vi "Read configuration.vi"(8 "error in":errorcluster, 11 "cfg group in":refnum<class "group node.lvclass">) -> (0 "error out":errorcluster, 2 "configuration":refnum<class "NISE_CEF_serializable configuration.lvclass">, 3 "cfg group out":refnum<class "group node.lvclass">)   [LabVIEW 2014, in "group node.lvclass"]
uses:
  group node.lvclass
  <vilib>/NI/Configuration Framework/serializable configuration/NISE_CEF_serializable configuration.lvclass
  group node.lvclass/group node.ctl
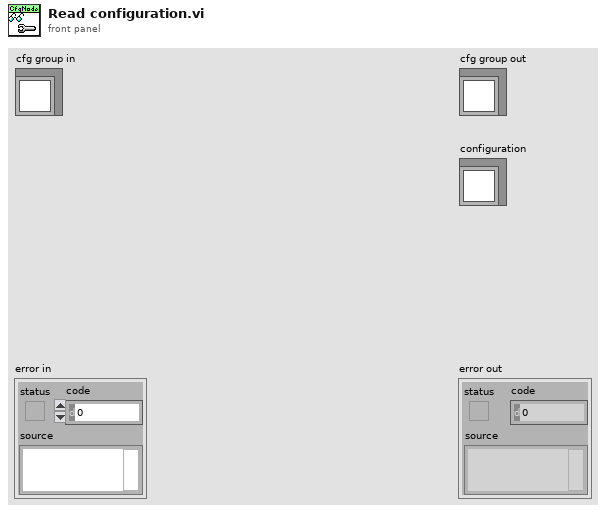
[diagram p1: front panel]
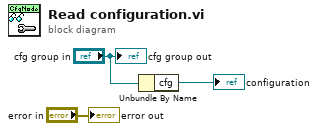
[diagram p0: block diagram]
diagram:
  n1 = Unbundle By Name("cfg group in") -> ("cfg"=→"configuration":refnum<class "group configuration.lvclass">)
  "error out" <- "error in"
  "cfg group out" <- "cfg group in"
